vi "Write Variance.vi"(8 "error in (no error)":errorcluster, 10 "Variance":dbl, 11 "Moving_Statistic in":refnum<class "Moving_Statistic.lvclass">) -> (0 "error out":errorcluster, 3 "Moving_Statistic out":refnum<class "Moving_Statistic.lvclass">)   [LabVIEW 2021, in "Moving_Statistic.lvclass"]
uses:
  Moving_Statistic.lvclass
  Moving_Statistic.lvclass/Moving_Statistic.ctl
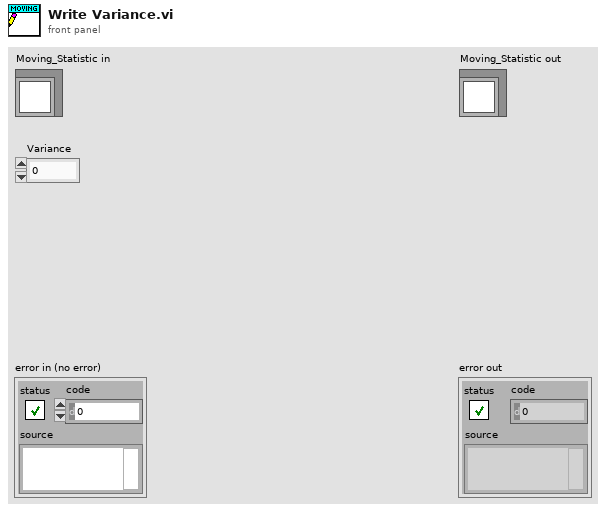
[diagram p1: front panel]
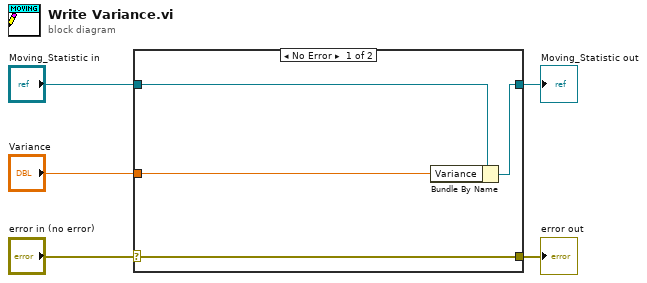
[diagram p0: block diagram]
diagram:
  n1 = case shown="No Error" "error in (no error)" {
    selector: "error in (no error)" -> [w9 w10]
    tunnel: [w9 w10] -> w4
    tunnel: [w7 w11] -> w2
    tunnel: "Moving_Statistic in" -> [w8 w11]
    tunnel: "Variance" -> [w6 _]
    frame No Error {
      n2 = Bundle By Name(cluster=w8, "Variance"=w6) -> (w7:refnum<class "Moving_Statistic.lvclass">)
    }
    frame Error {
    }
  }
  "error out" <- w4
  "Moving_Statistic out" <- w2
